vi "Move.vi"(7 "Shutter":T1={"Open command string"="+100\\s10\\n", "VISA"={"Timeout (ms)"=10000, "Resource Name"="COM1", "Baud Rate"=9600, "Data Bits"=8, "Parity"=0, "Stop Bits"=10, "Flow Control"=0}} {"VISA"."Flow Control" items=["None"=0, "XON/XOFF"=1, "RTS/CTS"=2, "DTR/DSR"=4]; "VISA"."Stop Bits" items=["1.0"=10, "1.5"=15, "2.0"=20]; "VISA"."Parity" items=["None", "Odd", "Even", "Mark", "Space"]}, 8 "error in (no error)":errorcluster, 11 "milliseconds to wait":u32) -> (0 "error out":errorcluster)   [LabVIEW 2017, in "Shutter.lvlib"]
uses:
  Shutter.lvlib
  Controls/Params.ctl
  Monochromator/Controls/VISA parameters.ctl
  Serial comms/Serial comms.lvlib
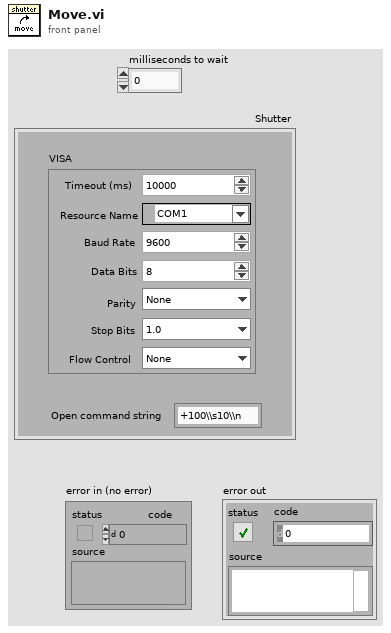
[diagram p1: front panel]
types:
  T1 = typedef "Shutter.lvlib/Params.ctl" = cluster{"Open command string":string, "VISA":T2}
  T2 = typedef "Serial comms.lvlib/VISA parameters.ctl" = cluster{"Timeout (ms)":u32, "Resource Name":refnum<visa-resource-name>, "Baud Rate":u32, "Data Bits":u16, "Parity":u16, "Stop Bits":u16, "Flow Control":u16}
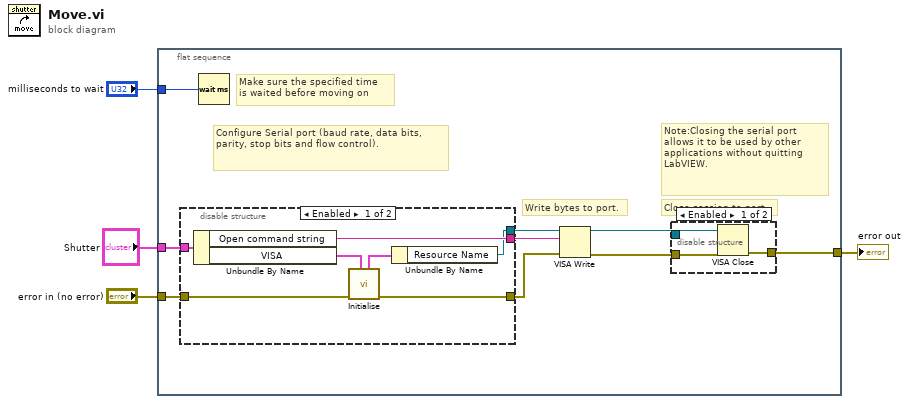
[diagram p0: block diagram]
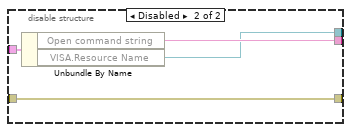
[diagram p3: hidden frame]
diagram:
  n1 = flat-sequence {
    tunnel: [w6] -> w4
    tunnel: "error in (no error)" -> [w10]
    tunnel: "milliseconds to wait" -> [w11]
    tunnel: "Shutter" -> [w8]
    frame #0 {
      # "Make sure the specified time \nis waited before moving on"
      # "Note:Closing the serial port allows it to be used by other applications without quitting LabVIEW."
      # "Close session to port."
      # "Configure Serial port (baud rate, data bits, parity, stop bits and flow control)."
      # "Write bytes to port."
      n2 = disable-structure shown="Enabled" {
        disable-tunnel: [w24 w28] -> w5
        disable-tunnel: w10 -> [w22 w25]
        disable-tunnel: [w21 w25] -> w9
        disable-tunnel: w8 -> [w20 w27]
        disable-tunnel: [w18 w26] -> w7
        frame Enabled {
          n3 = Unbundle By Name(w20) -> ("Open command string"=w24:string, "VISA"=w23:T2)
          n4 = call "Initialise.vi"("VISA parameters"=w23, "error in"=w22) -> ("error out"=w21:errorcluster, "VISA parameters out"=w19:T2)  [unwired: 8 in]
          n5 = Unbundle By Name(w19) -> ("Resource Name"=w18:refnum<visa-resource-name>)
        }
        frame Disabled {
          n6 = Unbundle By Name(w27) -> ("Open command string"=w28:string, "VISA.Resource Name"=w26:refnum<visa-resource-name>)
        }
      }
      n7 = Wait (ms)(milliseconds to wait=w11) -> ()  [unwired: 1 out]
      n8 = VISA Write(VISA resource name=w7, write buffer=w5, error in (no error)=w9) -> (VISA resource name out=w13:refnum<visa-resource-name>, error out=w12:errorcluster)  [unwired: 1 out]
      n9 = disable-structure shown="Enabled" {
        disable-tunnel: w13 -> [w16 _]
        disable-tunnel: w12 -> [w15 w17]
        disable-tunnel: [w14 w17] -> w6
        frame Enabled {
          n10 = VISA Close(VISA resource name=w16, error in (no error)=w15) -> (error out=w14:errorcluster)
        }
        frame Disabled {
        }
      }
    }
  }
  "error out" <- w4
